vi "MODBUS  SLAVE.vi"() -> (3 "values to write":u16[](array[numeric]) caption="待写入值")   [LabVIEW 2016]
uses:
  <vilib>/NI/Modbus Library/Data Model/Device Data Model.lvclass
  <vilib>/NI/Modbus Library/API/Wrapper/Create TCP Slave.vi
  <vilib>/NI/Modbus Library/API/slave/Modbus Slave.lvclass
  <vilib>/ptbypt/NI_PtbyPt.lvlib
  <vilib>/NI/Modbus Library/API/Wrapper/API Main.lvlib
panel:
  out "运行周期":u16[](array[numeric])
  in  "write operation starting address":u16=100 caption="写操作起始地址"
  out "单仪器启动命令":u16[](array[numeric])
  out "系统启动命令":u16[](array[numeric])
  in  "停止":bool
  out "register values":u16[](array[numeric]) caption="寄存器值"
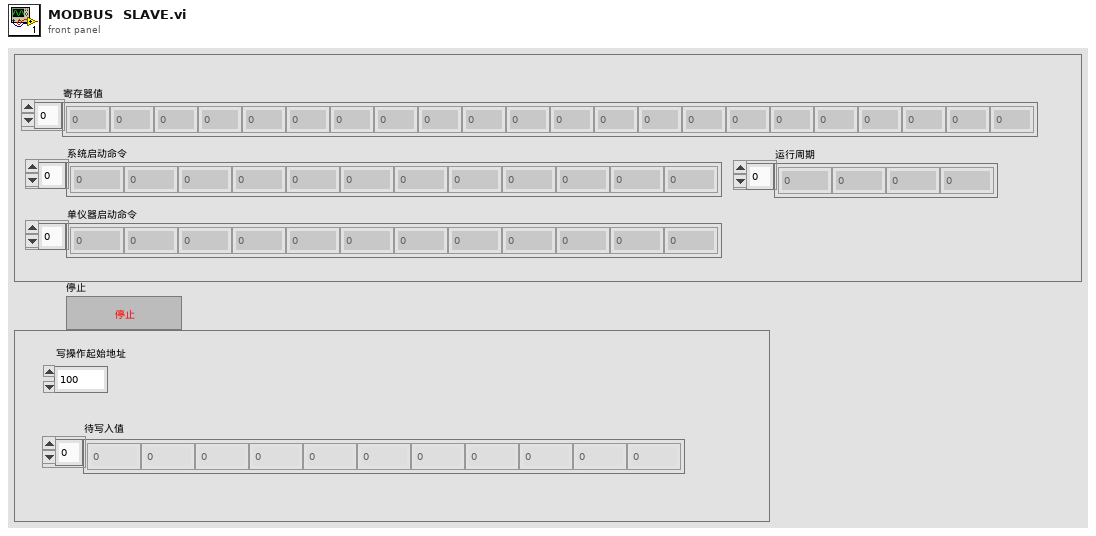
[diagram p1: front panel]
types:
  T1 = cluster{"测量模式":enum16{"水样测量", "标样核查", "零点核查", "跨度核查", "空白测试", "加标回收", "平行样", "校零", "校标"}}
  T2 = cluster{"站号":u16, "量程切换":enum32{"H", "L", "AUTO"}, "控制命令":enum16{"启动测量", "标样核查", "零点核查", "跨度核查", "空白测试", "平行样测试", "加标回收", "空白校准", "标样校准", "初始化（清洗）", "停止测试", "仪器重启", "校时", "模式设置", "测量间隔设置"}, "模式设置":enum16{"待机", "连续模式", "周期模式", "定点模式", "受控模式", "手动模式"}, "测量间隔":u16}
  T3 = cluster{"是否启用仪器":bool, "CODMn":cluster{"启动测量模式":cluster{"测量模式":enum16{"水样测量", "标样核查", "加标回收", "平行样", "校零", "校标"}}, "确定按钮":bool}, "启动模块":cluster{"氨氮":bool, "总磷":bool, "总氮":bool, "COD":bool}, "常规启动":bool, "直接启动":bool}
  T4 = cluster{"系统时间":timestamp, "工作状态":enum16{"空闲", "水样测试", "标样核查", "零点核查", "跨度核查", "空白测试", "平行样测试", "加标回收", "空白校准", "标样校准", "初始化（清洗）"}, "测量模式":enum16{"待机", "连续模式", "周期模式", "定点模式", "受控模式", "手动模式"}, "告警代码":u16, "故障代码":u16, "日志代码":u16, "软件版本":u16, "F0":sgl, "F1":sgl, "F2":sgl, "F3":sgl, "T":sgl, "H":sgl, "id":u16, "flowid":u16, "量程":u16, "总磷控温温度1":sgl, "营养盐控温温度2":sgl, "ADC":sgl}
  T5 = enum16{"空闲", "水样测试", "标样核查", "零点核查", "跨度核查", "空白测试", "平行样测试", "质控样", "空白校准", "标样校准", "加标回收"}
  T6 = cluster{"当前瓶号：":dbl, "平行样：":dbl, "留样瓶数：":dbl, "每瓶次数：":dbl, "每次留样：":dbl}
  T7 = enum16{"空闲", "水样测试", "标样核查", "零点核查", "跨度核查", "空白测试", "平行样测试", "加标回收", "空白校准", "标样校准", "初始化（清洗）"}
  T8 = enum32{"Bad", "Idle", "Run top level", "Running"}
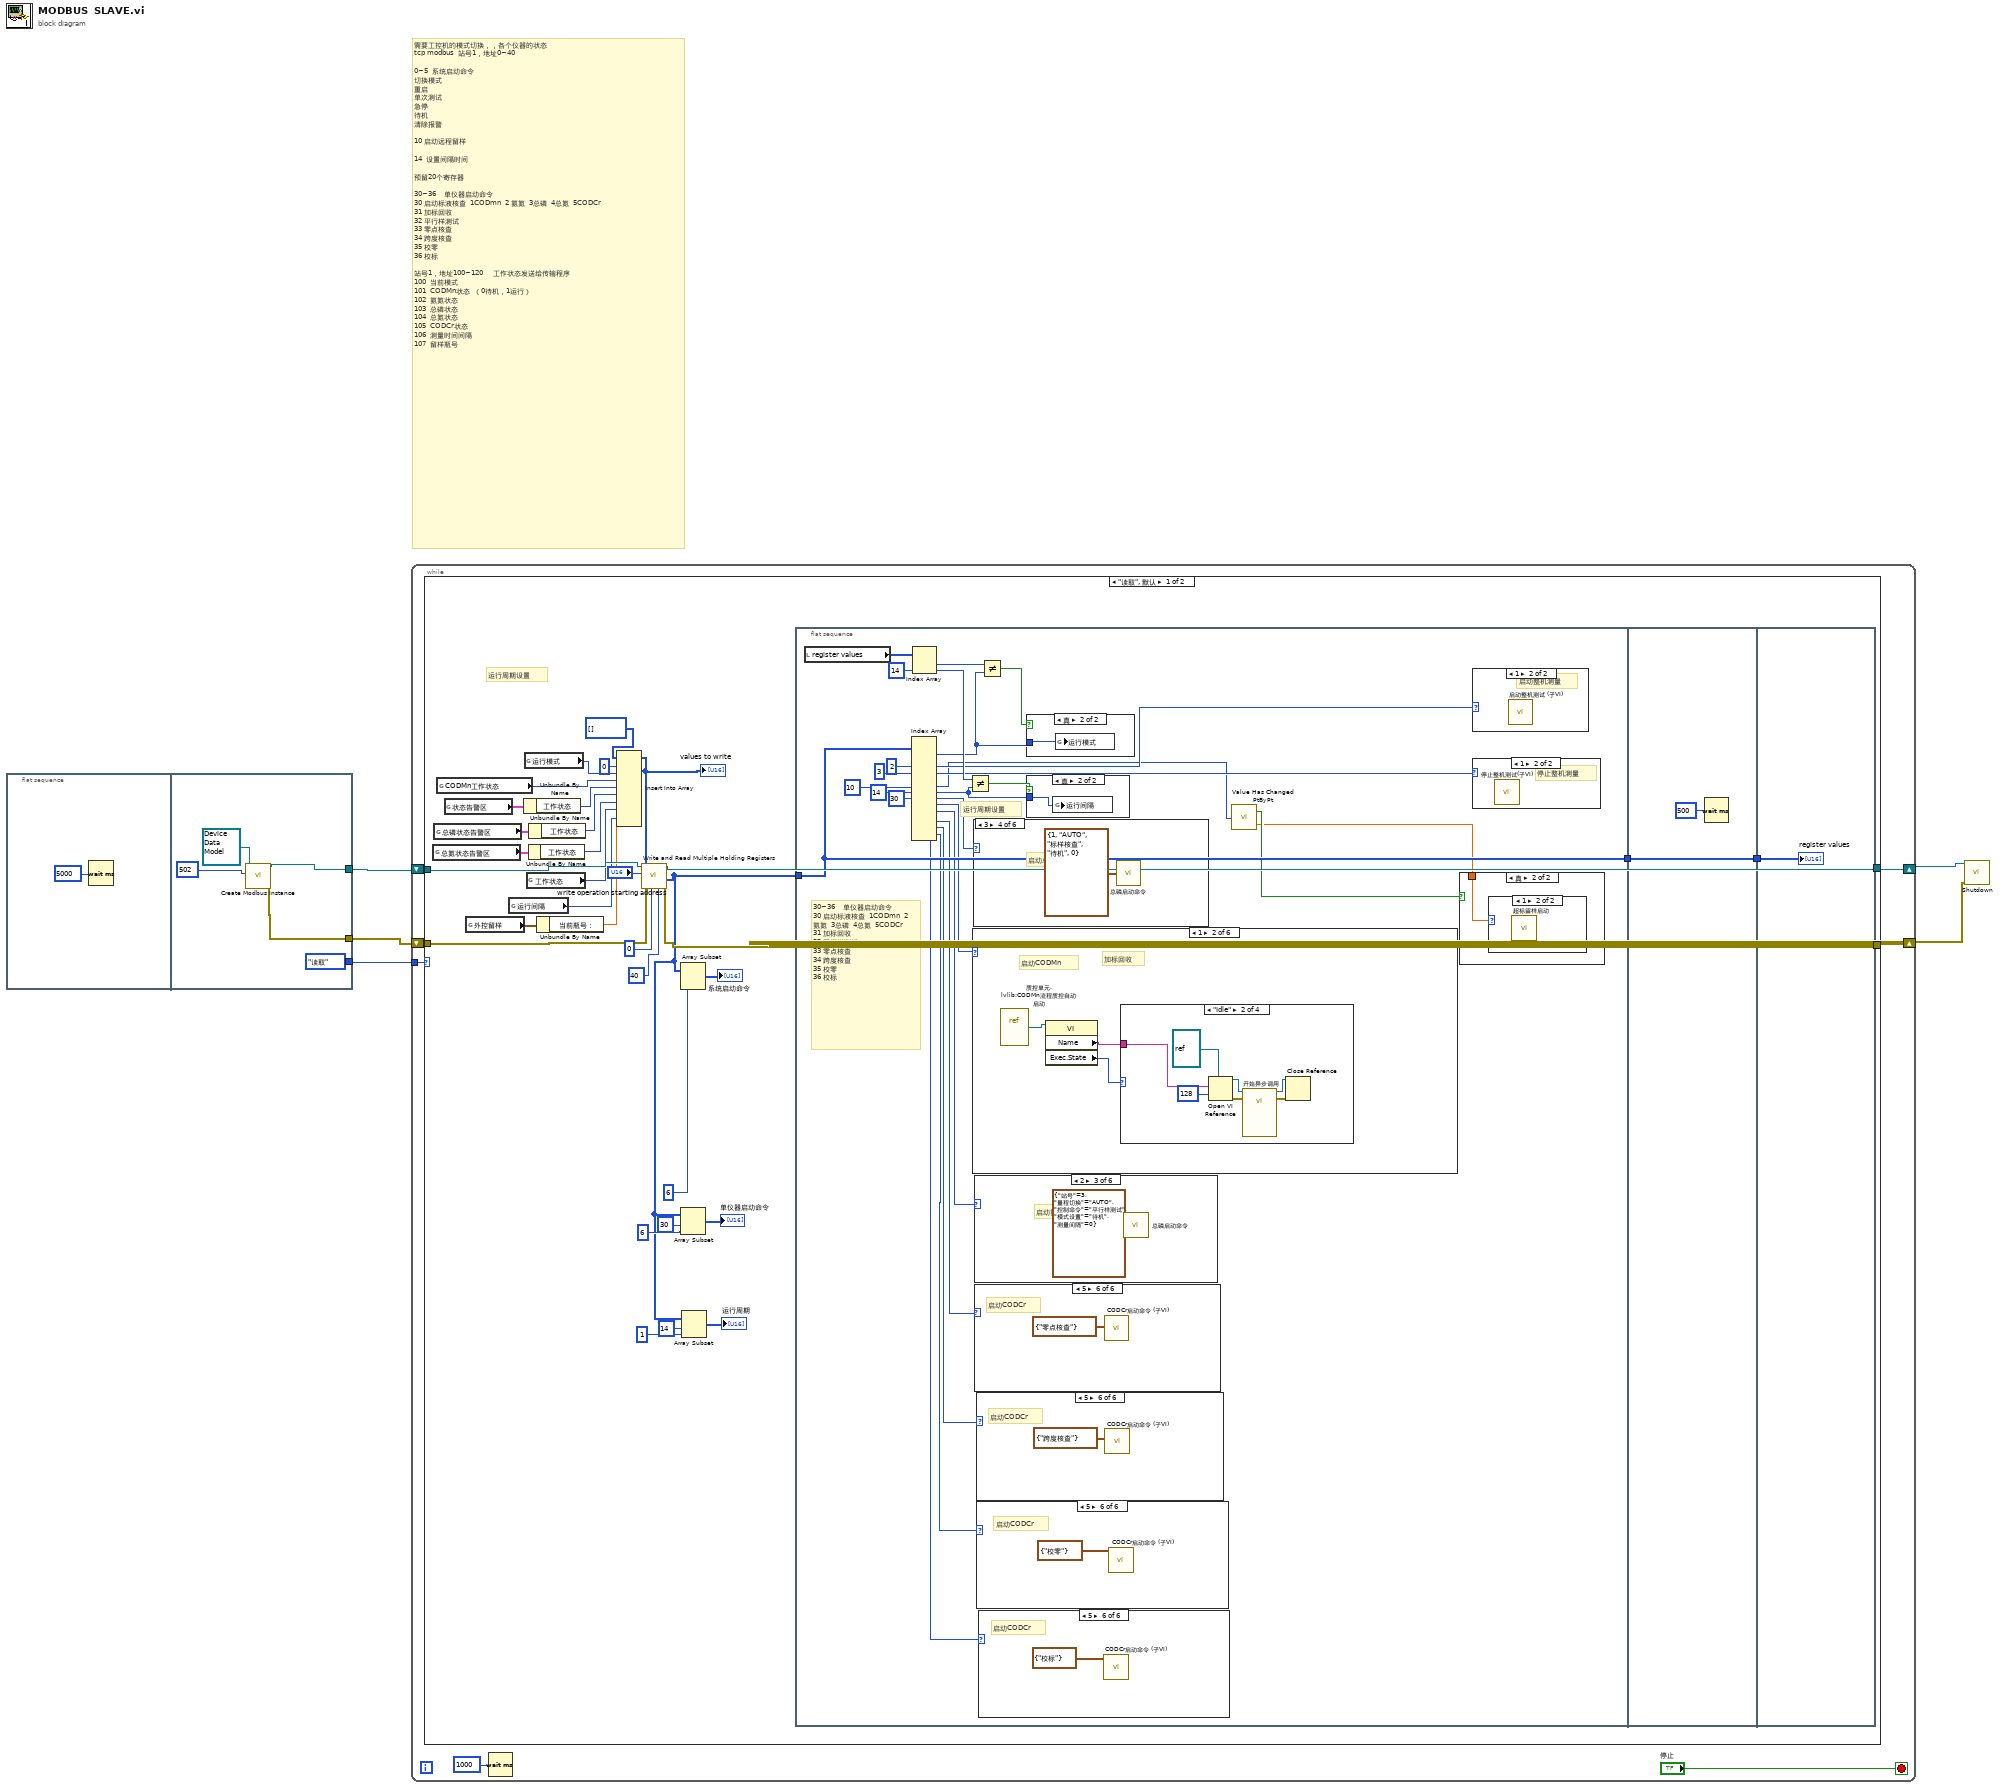
[diagram p0: block diagram]
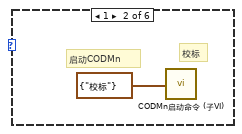
[diagram p5: hidden frame]
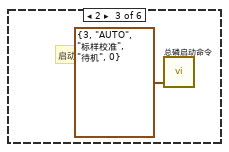
[diagram p6: hidden frame]
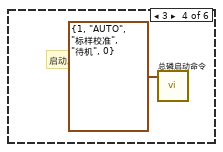
[diagram p7: hidden frame]
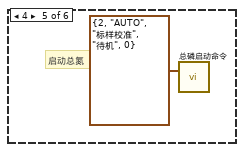
[diagram p8: hidden frame]
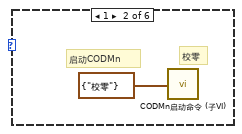
[diagram p10: hidden frame]
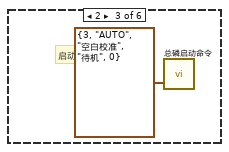
[diagram p11: hidden frame]
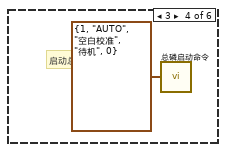
[diagram p12: hidden frame]
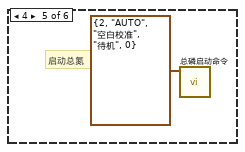
[diagram p13: hidden frame]
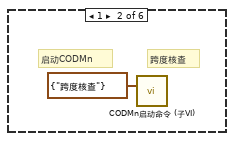
[diagram p15: hidden frame]
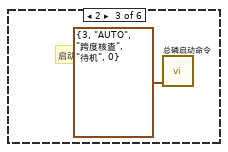
[diagram p16: hidden frame]
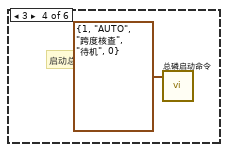
[diagram p17: hidden frame]
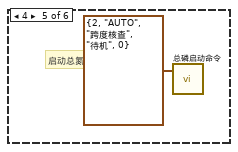
[diagram p18: hidden frame]
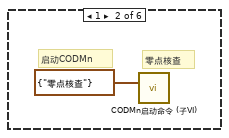
[diagram p20: hidden frame]
diagram:
  # "需要工控机的模式切换，，各个仪器的状态\ntcp modbus  站号1，地址0~40\n\n0~5  系统启动命令\n切换模式\n重启\n单次测试\n急停\n待机\n清除报警\n\n10 启动远程留样\n\n14  设置间隔时间\n\n预留20个寄存器\n\n30~36    单仪器启动命令\n30 启动标液核查  1CODmn  2 氨氮  3总磷  4总氮  5CODCr\n31 加标回收\n32 平行样测试\n33 零点核查\n34 跨度核查\n35 校零\n36 校标\n\n站号1，地址100~120     工作状态发送给传输程序\n100  当前模式\n101  CODMn状态  （0待机，1运行）\n102  氨氮状态\n103  总磷状态\n104  总氮状态\n105  CODCr状态\n106  测量时间间隔\n107  留样瓶号"
  n1 = flat-sequence {
    tunnel: [enum16{"读取", "写入"}."读取"] -> w5
    tunnel: [w9] -> w4
    tunnel: [w8] -> w3
    frame #0 {
      n2 = Wait (ms)(milliseconds to wait=u32 5000 ("等待时间（毫秒）")) -> ()  [unwired: 1 out]
    }
    frame #1 {
      n3 = call-poly <vilib>:"Create Modbus Instance.vi"("device data model"=refnum<class "Device Data Model.lvclass"> refnum, "port (502)"=u16 502) -> ("error out"=w9:errorcluster, "TCP slave instance"=w8:refnum<class "Modbus Slave.lvclass">)  [unwired: 8 in]
    }
  }
  n4 = while {
    shift-right: [w16] -> w2
    shift-left: w3 -> [w18]
    shift-right: [w12] -> w1
    shift-left: w4 -> [w17]
    tunnel: w5 -> [w13]
    stop <- "停止" stop-if-true
    n5 = case shown="\"读取\", 默认" w13 {
      tunnel: w18 -> [w47 w164]
      tunnel: w17 -> [w46 w163]
      tunnel: [w42 w164] -> w16
      tunnel: [w43 w163] -> w12
      frame "读取", Default {
        # "运行周期设置"
        n6 = global read "VAR总磷全局变量.vi" "总氮状态告警区"() -> (w25:T4)
        n7 = global read "VAR总磷全局变量.vi" "总磷状态告警区"() -> (w27:T4)
        n8 = global read "COD测量模式全局.vi" "CODMn工作状态"() -> (w23:T5)
        n9 = global read "VAR氨氮全局变量.vi" "状态告警区"() -> (w29:T4)
        n10 = global read "超标留样全局.vi" "外控留样"() -> (w20:T6)
        n11 = global read "系统设置全局变量.vi" "运行间隔"() -> (w21:i16)
        n12 = Unbundle By Name(w29) -> ("工作状态"=w28:T7)
        n13 = global read "系统设置全局变量.vi" "运行模式"() -> (w39:enum16{"维护模式", "常规模式", "应急模式", "质控模式"})
        n14 = global read "CODcr全局变量.vi" "工作状态"() -> (w22:T7)
        n15 = Unbundle By Name(w25) -> ("工作状态"=w24:T7)
        n16 = Unbundle By Name(w27) -> ("工作状态"=w26:T7)
        n17 = Unbundle By Name(w20) -> ("当前瓶号："=w19:dbl)
        n18 = Insert Into Array(array=u16[] [] ("values to write"), index=0 ("索引"), new element #1=w39, new element #2=w23, new element #3=w28, new element #4=w26, new element #5=w24, new element #6=w22, new element #7=w21, new element #8=w19) -> (w37:u16[])
        "values to write" <- w37
        n19 = call-dynamic "Write and Read Multiple Holding Registers.vi"("read count"=u16 40 ("number of holding registers"), "read starting address"=u16 0 ("starting address"), "error in"=w46, "write values"=w37, "write starting address"="write operation starting address", "Modbus instance in"=w47) -> ("error out"=w43:errorcluster, "read values"=w32:u16[], "Modbus instance out"=w42:refnum<class "Modbus Slave.lvclass">)  [unwired: 3 in]
        n20 = Array Subset(array=w32, length=6 ("长度")) -> (→"系统启动命令":u16[])  [unwired: 1 in]
        n21 = Array Subset(array=w32, index=30 ("索引"), length=6 ("长度")) -> (→"单仪器启动命令":u16[])
        n22 = Array Subset(array=w32, index=14 ("索引"), length=1 ("长度")) -> (→"运行周期":u16[])
        n23 = flat-sequence {
          tunnel: w32 -> [w77]
          tunnel: [w77] -> w31
          tunnel: w31 -> [w160]
          tunnel: [w160] -> w30
          tunnel: w30 -> [w162]
          frame #0 {
            # "运行周期设置"
            # "30~36    单仪器启动命令\n30 启动标液核查  1CODmn  2 氨氮  3总磷  4总氮  5CODCr\n31 加标回收\n32 平行样测试\n33 零点核查\n34 跨度核查\n35 校零\n36 校标"
            n24 = local read "register values"() -> (w76:u16[])
            n25 = Index Array(array=w77, index #3=2 ("索引"), index #4=3 ("索引"), index #6=10 ("索引"), index #7=14 ("索引"), index #8=30 ("索引")) -> (element #1=w64:u16, element #3=w65:u16, element #4=w66:u16, element #6=w54:u16, element #7=w67:u16, element #8=w62:u16, element #9=w61:u16, element #10=w60:u16, element #11=w59:u16, element #12=w58:u16, element #13=w57:u16, element #14=w56:u16)  [unwired: 9 in, 2 out]
            n26 = Index Array(array=w76, index #2=14 ("索引")) -> (element #1=w75:u16, element #2=w72:u16)  [unwired: 1 in]
            n27 = Not Equal?(x=w72, y=w67) -> (x != y?=w71:bool)
            n28 = case shown="1" w61 {
              frame 0, Default {
              }
              frame 1 {
                # "加标回收"
                # "启动CODMn"
                n29 = vi-ref "质控单元.lvlib:CODMn流程质控自动启动.vi"() -> (w104:refnum<vi>)
                n30 = property class="VI"(reference=w104) -> ("Name"=w106:string, "Exec.State"=w105:T8)  [unwired: 1 in, 2 out]
                n31 = case shown="\"Idle\"" w105 {
                  tunnel: w106 -> [_ w109 _ _]
                  frame "Bad", Default {
                  }
                  frame "Idle" {
                    n32 = Open VI Reference(type specifier VI Refnum (for type only)=refnum<vi> refnum ("类型说明符VI引用句柄（仅用于类型）"), vi path=w109, options=128 ("选项")) -> (vi reference=w113:refnum<vi>, error out=w108:errorcluster)  [unwired: 3 in]
                    n33 = call-by-ref "开始异步调用"(reference=w113, error in=w108) -> (reference out=w112:refnum<vi>, error out=w107:errorcluster)  [unwired: 12 in]
                    n34 = Close Reference(reference=w112, error in (no error)=w107) -> ()  [unwired: 1 out]
                  }
                  frame "Run top level" {
                  }
                  frame "Running" {
                  }
                }
              }
              frame 2 {
                # "启动氨氮"
                n35 = vi-ref "质控单元.lvlib:氨氮流程质控自动启动.vi"() -> (w116:refnum<vi>)
                n36 = property class="VI"(reference=w116) -> ("Name"=w114:string, "Exec.State"=w115:T8)  [unwired: 1 in, 2 out]
                n37 = case shown="\"Idle\"" w115 {
                  tunnel: w114 -> [_ w119 _ _]
                  frame "Bad", Default {
                  }
                  frame "Idle" {
                    n38 = Open VI Reference(type specifier VI Refnum (for type only)=refnum<vi> refnum ("类型说明符VI引用句柄（仅用于类型）"), vi path=w119, options=128 ("选项")) -> (vi reference=w123:refnum<vi>, error out=w118:errorcluster)  [unwired: 3 in]
                    n39 = call-by-ref "开始异步调用"(reference=w123, error in=w118) -> (reference out=w122:refnum<vi>, error out=w117:errorcluster)  [unwired: 12 in]
                    n40 = Close Reference(reference=w122, error in (no error)=w117) -> ()  [unwired: 1 out]
                  }
                  frame "Run top level" {
                  }
                  frame "Running" {
                  }
                }
              }
              frame 3 {
                # "启动总磷"
                n41 = vi-ref "质控单元.lvlib:总磷总氮流程质控自动启动.vi"() -> (w126:refnum<vi>)
                n42 = property class="VI"(reference=w126) -> ("Name"=w125:string, "Exec.State"=w124:T8)  [unwired: 1 in, 2 out]
                n43 = case shown="\"Idle\"" w124 {
                  tunnel: w125 -> [_ w133 _ _]
                  frame "Bad", Default {
                  }
                  frame "Idle" {
                    n44 = Bundle By Name(cluster=T3 {"是否启用仪器"=FALSE, "CODMn"={"启动测量模式"={"测量模式"=enum."水样测量"}, "确定按钮"=FALSE}, "启动模块"={"氨氮"=FALSE, "总磷"=FALSE, "总氮"=FALSE, "COD"=FALSE}, "常规启动"=FALSE, "直接启动"=FALSE} ("参数"), "启动模块.总磷"=TRUE, "启动模块.总氮"=FALSE) -> (w129:T3)
                    n45 = Open VI Reference(type specifier VI Refnum (for type only)=refnum<vi> refnum ("类型说明符VI引用句柄（仅用于类型）"), vi path=w133, options=128 ("选项")) -> (vi reference=w137:refnum<vi>, error out=w131:errorcluster)  [unwired: 3 in]
                    n46 = call-by-ref "开始异步调用"(reference=w137, error in=w131, "参数"=w129) -> (reference out=w136:refnum<vi>, error out=w132:errorcluster)  [unwired: 11 in]
                    n47 = Close Reference(reference=w136, error in (no error)=w132) -> ()  [unwired: 1 out]
                  }
                  frame "Run top level" {
                  }
                  frame "Running" {
                  }
                }
              }
              frame 4 {
                # "启动总氮"
                n48 = vi-ref "质控单元.lvlib:总磷总氮流程质控自动启动.vi"() -> (w140:refnum<vi>)
                n49 = property class="VI"(reference=w140) -> ("Name"=w139:string, "Exec.State"=w138:T8)  [unwired: 1 in, 2 out]
                n50 = case shown="\"Idle\"" w138 {
                  tunnel: w139 -> [_ w147 _ _]
                  frame "Bad", Default {
                  }
                  frame "Idle" {
                    n51 = Bundle By Name(cluster=T3 {"是否启用仪器"=FALSE, "CODMn"={"启动测量模式"={"测量模式"=enum."水样测量"}, "确定按钮"=FALSE}, "启动模块"={"氨氮"=FALSE, "总磷"=FALSE, "总氮"=FALSE, "COD"=FALSE}, "常规启动"=FALSE, "直接启动"=FALSE} ("参数"), "启动模块.总磷"=FALSE, "启动模块.总氮"=TRUE) -> (w143:T3)
                    n52 = Open VI Reference(type specifier VI Refnum (for type only)=refnum<vi> refnum ("类型说明符VI引用句柄（仅用于类型）"), vi path=w147, options=128 ("选项")) -> (vi reference=w151:refnum<vi>, error out=w145:errorcluster)  [unwired: 3 in]
                    n53 = call-by-ref "开始异步调用"(reference=w151, error in=w145, "参数"=w143) -> (reference out=w150:refnum<vi>, error out=w146:errorcluster)  [unwired: 11 in]
                    n54 = Close Reference(reference=w150, error in (no error)=w146) -> ()  [unwired: 1 out]
                  }
                  frame "Run top level" {
                  }
                  frame "Running" {
                  }
                }
              }
              frame 5 {
                # "启动CODCr"
                n55 = call "CODCr启动命令 (子VI).vi"("启动测量模式"=T1 {"测量模式"=enum."加标回收"}) -> ()  [unwired: 11 in]
              }
            }
            n56 = case shown="3" w62 {
              frame 0, Default {
              }
              frame 1 {
                # "启动标液核查"
                # "启动CODMn"
                n57 = call "CODMn启动命令 (子VI).vi"("启动测量模式"=T1 {"测量模式"=enum."标样核查"}) -> ()  [unwired: 11 in]
              }
              frame 2 {
                # "启动氨氮"
                n58 = call "总磷启动命令.vi"("参数"=T2 {"站号"=3, "量程切换"=enum."AUTO", "控制命令"=enum."标样核查", "模式设置"=enum."待机", "测量间隔"=0}) -> ()  [unwired: 10 in, 1 out]
              }
              frame 3 {
                # "启动总磷"
                n59 = call "总磷启动命令.vi"("参数"=T2 {"站号"=1, "量程切换"=enum."AUTO", "控制命令"=enum."标样核查", "模式设置"=enum."待机", "测量间隔"=0}) -> ()  [unwired: 10 in, 1 out]
              }
              frame 4 {
                # "启动总氮"
                n60 = call "总磷启动命令.vi"("参数"=T2 {"站号"=2, "量程切换"=enum."AUTO", "控制命令"=enum."标样核查", "模式设置"=enum."待机", "测量间隔"=0}) -> ()  [unwired: 10 in, 1 out]
              }
              frame 5 {
                # "启动CODCr"
                n61 = call "CODCr启动命令 (子VI).vi"("启动测量模式"=T1 {"测量模式"=enum."标样核查"}) -> ()  [unwired: 11 in]
              }
            }
            n62 = case shown="2" w60 {
              frame 0, Default {
              }
              frame 1 {
                # "平行样测试"
                # "启动CODMn"
                n63 = call "CODMn启动命令 (子VI).vi"("启动测量模式"=T1 {"测量模式"=enum."平行样"}) -> ()  [unwired: 11 in]
              }
              frame 2 {
                # "启动氨氮"
                n64 = call "总磷启动命令.vi"("参数"=T2 {"站号"=3, "量程切换"=enum."AUTO", "控制命令"=enum."平行样测试", "模式设置"=enum."待机", "测量间隔"=0}) -> ()  [unwired: 10 in, 1 out]
              }
              frame 3 {
                # "启动总磷"
                n65 = call "总磷启动命令.vi"("参数"=T2 {"站号"=1, "量程切换"=enum."AUTO", "控制命令"=enum."平行样测试", "模式设置"=enum."待机", "测量间隔"=0}) -> ()  [unwired: 10 in, 1 out]
              }
              frame 4 {
                # "启动总氮"
                n66 = call "总磷启动命令.vi"("参数"=T2 {"站号"=2, "量程切换"=enum."AUTO", "控制命令"=enum."平行样测试", "模式设置"=enum."待机", "测量间隔"=0}) -> ()  [unwired: 10 in, 1 out]
              }
              frame 5 {
                # "启动CODCr"
                n67 = call "CODCr启动命令 (子VI).vi"("启动测量模式"=T1 {"测量模式"=enum."平行样"}) -> ()  [unwired: 11 in]
              }
            }
            n68 = case shown="5" w59 {
              frame 0, Default {
              }
              frame 1 {
                # "零点核查"
                # "启动CODMn"
                n69 = call "CODMn启动命令 (子VI).vi"("启动测量模式"=T1 {"测量模式"=enum."零点核查"}) -> ()  [unwired: 11 in]
              }
              frame 2 {
                # "启动氨氮"
                n70 = call "总磷启动命令.vi"("参数"=T2 {"站号"=3, "量程切换"=enum."AUTO", "控制命令"=enum."零点核查", "模式设置"=enum."待机", "测量间隔"=0}) -> ()  [unwired: 10 in, 1 out]
              }
              frame 3 {
                # "启动总磷"
                n71 = call "总磷启动命令.vi"("参数"=T2 {"站号"=1, "量程切换"=enum."AUTO", "控制命令"=enum."零点核查", "模式设置"=enum."待机", "测量间隔"=0}) -> ()  [unwired: 10 in, 1 out]
              }
              frame 4 {
                # "启动总氮"
                n72 = call "总磷启动命令.vi"("参数"=T2 {"站号"=2, "量程切换"=enum."AUTO", "控制命令"=enum."零点核查", "模式设置"=enum."待机", "测量间隔"=0}) -> ()  [unwired: 10 in, 1 out]
              }
              frame 5 {
                # "启动CODCr"
                n73 = call "CODCr启动命令 (子VI).vi"("启动测量模式"=T1 {"测量模式"=enum."零点核查"}) -> ()  [unwired: 11 in]
              }
            }
            n74 = case shown="5" w58 {
              frame 0, Default {
              }
              frame 1 {
                # "跨度核查"
                # "启动CODMn"
                n75 = call "CODMn启动命令 (子VI).vi"("启动测量模式"=T1 {"测量模式"=enum."跨度核查"}) -> ()  [unwired: 11 in]
              }
              frame 2 {
                # "启动氨氮"
                n76 = call "总磷启动命令.vi"("参数"=T2 {"站号"=3, "量程切换"=enum."AUTO", "控制命令"=enum."跨度核查", "模式设置"=enum."待机", "测量间隔"=0}) -> ()  [unwired: 10 in, 1 out]
              }
              frame 3 {
                # "启动总磷"
                n77 = call "总磷启动命令.vi"("参数"=T2 {"站号"=1, "量程切换"=enum."AUTO", "控制命令"=enum."跨度核查", "模式设置"=enum."待机", "测量间隔"=0}) -> ()  [unwired: 10 in, 1 out]
              }
              frame 4 {
                # "启动总氮"
                n78 = call "总磷启动命令.vi"("参数"=T2 {"站号"=2, "量程切换"=enum."AUTO", "控制命令"=enum."跨度核查", "模式设置"=enum."待机", "测量间隔"=0}) -> ()  [unwired: 10 in, 1 out]
              }
              frame 5 {
                # "启动CODCr"
                n79 = call "CODCr启动命令 (子VI).vi"("启动测量模式"=T1 {"测量模式"=enum."跨度核查"}) -> ()  [unwired: 11 in]
              }
            }
            n80 = case shown="5" w57 {
              frame 0, Default {
              }
              frame 1 {
                # "校零"
                # "启动CODMn"
                n81 = call "CODMn启动命令 (子VI).vi"("启动测量模式"=T1 {"测量模式"=enum."校零"}) -> ()  [unwired: 11 in]
              }
              frame 2 {
                # "启动氨氮"
                n82 = call "总磷启动命令.vi"("参数"=T2 {"站号"=3, "量程切换"=enum."AUTO", "控制命令"=enum."空白校准", "模式设置"=enum."待机", "测量间隔"=0}) -> ()  [unwired: 10 in, 1 out]
              }
              frame 3 {
                # "启动总磷"
                n83 = call "总磷启动命令.vi"("参数"=T2 {"站号"=1, "量程切换"=enum."AUTO", "控制命令"=enum."空白校准", "模式设置"=enum."待机", "测量间隔"=0}) -> ()  [unwired: 10 in, 1 out]
              }
              frame 4 {
                # "启动总氮"
                n84 = call "总磷启动命令.vi"("参数"=T2 {"站号"=2, "量程切换"=enum."AUTO", "控制命令"=enum."空白校准", "模式设置"=enum."待机", "测量间隔"=0}) -> ()  [unwired: 10 in, 1 out]
              }
              frame 5 {
                # "启动CODCr"
                n85 = call "CODCr启动命令 (子VI).vi"("启动测量模式"=T1 {"测量模式"=enum."校零"}) -> ()  [unwired: 11 in]
              }
            }
            n86 = case shown="5" w56 {
              frame 0, Default {
              }
              frame 1 {
                # "校标"
                # "启动CODMn"
                n87 = call "CODMn启动命令 (子VI).vi"("启动测量模式"=T1 {"测量模式"=enum."校标"}) -> ()  [unwired: 11 in]
              }
              frame 2 {
                # "启动氨氮"
                n88 = call "总磷启动命令.vi"("参数"=T2 {"站号"=3, "量程切换"=enum."AUTO", "控制命令"=enum."标样校准", "模式设置"=enum."待机", "测量间隔"=0}) -> ()  [unwired: 10 in, 1 out]
              }
              frame 3 {
                # "启动总磷"
                n89 = call "总磷启动命令.vi"("参数"=T2 {"站号"=1, "量程切换"=enum."AUTO", "控制命令"=enum."标样校准", "模式设置"=enum."待机", "测量间隔"=0}) -> ()  [unwired: 10 in, 1 out]
              }
              frame 4 {
                # "启动总氮"
                n90 = call "总磷启动命令.vi"("参数"=T2 {"站号"=2, "量程切换"=enum."AUTO", "控制命令"=enum."标样校准", "模式设置"=enum."待机", "测量间隔"=0}) -> ()  [unwired: 10 in, 1 out]
              }
              frame 5 {
                # "启动CODCr"
                n91 = call "CODCr启动命令 (子VI).vi"("启动测量模式"=T1 {"测量模式"=enum."校标"}) -> ()  [unwired: 11 in]
              }
            }
            n92 = Not Equal?(x=w75, y=w64) -> (x != y?=w74:bool)
            n93 = case shown="真" w74 {
              tunnel: w64 -> [_ w159]
              frame False {
              }
              frame True {
                n94 = global write "系统设置全局变量.vi" "运行模式"(w159) -> ()
              }
            }
            n95 = case shown="真" w71 {
              tunnel: w67 -> [_ w158]
              frame False {
              }
              frame True {
                n96 = global write "系统设置全局变量.vi" "运行间隔"(w158) -> ()
              }
            }
            n97 = call <vilib>:"Value Has Changed PtByPt.vi"("input data point"=w54) -> ("has changed"=w53:bool, "output data point"=w52:dbl)  [unwired: 1 in]
            n98 = case shown="真" w53 {
              tunnel: w52 -> [_ w78]
              frame False {
              }
              frame True {
                n99 = case shown="1" w78 {
                  frame 0, Default {
                  }
                  frame 1 {
                    n100 = call "超标留样启动.vi"() -> ()  [unwired: 11 in, 1 out]
                  }
                }
              }
            }
            n101 = case shown="1" w66 {
              frame 0, Default {
              }
              frame 1 {
                # "停止整机测量"
                n102 = call "停止整机测试(子VI).vi"() -> ()  [unwired: 12 in]
              }
            }
            n103 = case shown="1" w65 {
              frame 0, Default {
              }
              frame 1 {
                # "启动整机测量"
                n104 = call "启动整机测试 (子VI).vi"() -> ()  [unwired: 12 in]
              }
            }
          }
          frame #1 {
            n105 = Wait (ms)(milliseconds to wait=u32 500 ("等待时间（毫秒）")) -> ()  [unwired: 1 out]
          }
          frame #2 {
            "register values" <- w162
          }
        }
      }
      frame "写入" {
      }
    }
    n106 = Wait (ms)(milliseconds to wait=u32 1000 ("等待时间（毫秒）")) -> ()  [unwired: 1 out]
  }
  n107 = call-dynamic "Shutdown.vi"("error in"=w1, "Modbus slave in"=w2) -> ()  [unwired: 9 in, 1 out]
